vi "GET CUSTOM ITEM.vi"(11 "REFERENCES":T1) -> ()   [LabVIEW 2019]
uses:
  Controls/References Cluster.ctl
  <vilib>/userDefined/High Color/IMAQdx.ctl
  Controls/Custom Calendar/Custom Calendar.xctl
types:
  T1 = typedef "References Cluster.ctl" = cluster{"MAIN PAGES":refnum<vi>, "ADD/EDIT ITEM REFERENCES":cluster{"Identifier":refnum<vi>, "BYU ICN #":refnum<vi>, "Item Description":refnum<vi>, "Comments":refnum<vi>, "Checked Out Date":refnum<vi>, "Due Date":refnum<vi>, "Check Out Location":refnum<vi>, "Reminder Count":refnum<vi>, "Most Recent Reminder Date":refnum<vi>, "BYU ID #":refnum<vi>, "Building/Room":refnum<vi>, "Location in Room":refnum<vi>, "Manual":refnum<vi>, "Manufacturer":refnum<vi>, "Model #":refnum<vi>, "Serial #":refnum<vi>, "Date Acquired":refnum<vi>, "ADD/EDIT ITEM LABEL":refnum<vi>, "ARCHIVE ITEM":refnum<vi>, "Archive Item Inputs":refnum<vi>, "Reminder Notes":refnum<vi>}, "ADD/EDIT USER REFERENCES":cluster{"BYU ID # (##-###-####)":refnum<vi>, "First Name":refnum<vi>, "Last Name":refnum<vi>, "Phone Number (###-###-####)":refnum<vi>, "Email":refnum<vi>, "Department":refnum<vi>, "Graduation Status":refnum<vi>, "Anticipated Graduation Year":refnum<vi>, "Credit Score":refnum<vi>, "Date Added":refnum<vi>, "Graduation Clearance Date":refnum<vi>, "Picture File Name":refnum<vi>, "ADD/EDIT USER LABEL":refnum<vi>, "Department Map":refnum<vi>, "Status Map":refnum<vi>, "Anticipated Graduation Year Map":refnum<vi>, "User Agreement":refnum<vi>, "User Comments":refnum<vi>, "Camera":refnum<vi>}, "RETURN ITEM REFERENCES":cluster{"Item or Person:":refnum<vi>, "Search Return Results":refnum<vi>, "What are you searching for?":refnum<vi>}, "SEARCH DATABASE REFERENCES":cluster{"What to Search For:":refnum<vi>, "Where to Search":refnum<vi>, "Column to Search In":refnum<vi>, "Column to Sort By":refnum<vi>, "Search Database Results":refnum<vi>, "Inventory Column Selector":refnum<vi>, "User Column Selector":refnum<vi>, "Inventory Archive Column Selector":refnum<vi>, "User Archive Column Selector":refnum<vi>, "Sales Tracking Column Selector":refnum<vi>, "Checked In Archive Column Selector":refnum<vi>, "Restore User":refnum<vi>, "Date Range":refnum<vi>, "Dates Less Than":refnum<vi>, "Dates Greater Than":refnum<vi>, "Search Print Receipt":refnum<vi>, "Edit Sale Description":refnum<vi>}, "USER ITEMS REFERENCES":cluster{"USER'S INFORMATION":refnum<vi>, "User's Checked Out Items":refnum<vi>, "User Info Comments":refnum<vi>, "SEE USER INFO COMMENTS":refnum<vi>}, "EDIT ITEMS REFERENCES":cluster{"New Check Out Location":refnum<vi>, "Items to Edit":refnum<vi>, "Edit Items Due Date":refnum<vi>, "New Reminder Notes":refnum<vi>, "New Item Description":refnum<vi>}, "CHECK OUT ITEMS REFERENCES":cluster{"Enter Item:":refnum<vi>, "Check Out Items Due Date":refnum<vi>, "Check Out Location":refnum<vi>, "Items to be Checked Out":refnum<vi>, "Possible Items":refnum<vi>}, "TRANSFER ITEMS REFERENCES":cluster{"Search Parameter":refnum<vi>, "What to Match":refnum<vi>, "Matching Individuals":refnum<vi>, "Items to be Transferred":refnum<vi>}, "SETTINGS REFERENCES":cluster{"PSC Database Settings":refnum<vi>, "PSC Sales Item Spreadsheet":refnum<vi>}, "PSC SALES REFERENCES":cluster{"BYU ID CARD #":refnum<vi>, "Sale Description":refnum<vi>, "Scan or Enter Item Name":refnum<vi>, "Items to be Sold":refnum<vi>, "Grand Total":refnum<vi>, "Item List":refnum<vi>}}
  T2 = cluster{"BYU ID CARD #":refnum<vi>, "Sale Description":refnum<vi>, "Scan or Enter Item Name":refnum<vi>, "Items to be Sold":refnum<vi>, "Grand Total":refnum<vi>, "Item List":refnum<vi>}
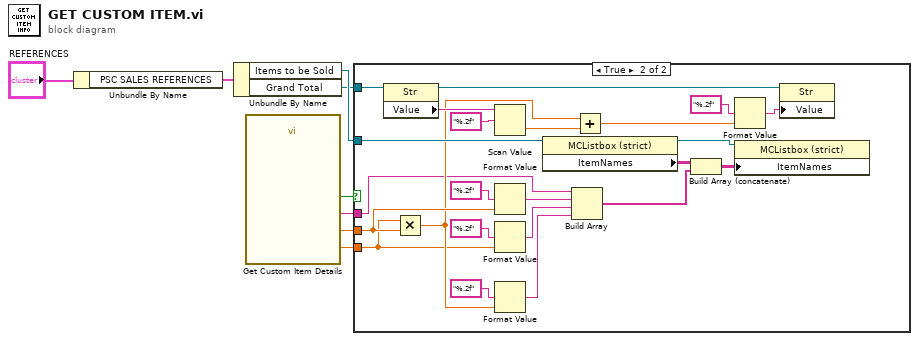
[diagram p0: block diagram]
diagram:
  n1 = Unbundle By Name("REFERENCES") -> ("PSC SALES REFERENCES"=w7:T2)
  n2 = Unbundle By Name(w7) -> ("Items to be Sold"=w5:refnum<vi>, "Grand Total"=w4:refnum<vi>)
  n3 = call "Get Custom Item Details"() -> ("Price"=w1:dbl, "Quantity"=w3:dbl, "Name"=w2:string, "OK"=w6:bool)  [unwired: 15 in, 1 out]
  n4 = case shown="True" w6 {
    tunnel: w3 -> [_ w26]
    tunnel: w5 -> [_ w31]
    tunnel: w4 -> [_ w30]
    tunnel: w2 -> [_ w12]
    tunnel: w1 -> [_ w11]
    frame False {
    }
    frame True {
      n5 = property class="Str"(reference=w30) -> (reference out=w20:refnum<vi>, "Value"=w24:string)  [unwired: 1 in, 1 out]
      n6 = Multiply(x=w11, y=w26) -> (x*y=w13:dbl)
      n7 = Scan Value(string=w24, format string="%.2f") -> (value=w23:dbl)  [unwired: 1 in, 1 out]
      n8 = Format Value(format string="%.2f", value (0)=w26) -> (output string=w27:string)  [unwired: 1 in]
      n9 = Format Value(format string="%.2f", value (0)=w11) -> (output string=w9:string)  [unwired: 1 in]
      n10 = Format Value(format string="%.2f", value (0)=w13) -> (output string=w17:string)  [unwired: 1 in]
      n11 = property class="MCListbox (strict)"(reference=w31) -> (reference out=w15:refnum<vi>, "ItemNames"=w29:string[][])  [unwired: 1 in, 1 out]
      n12 = Build Array(w12, w27, w9, w17) -> (w16:string[])
      n13 = Add(x=w13, y=w23) -> (x+y=w21:dbl)
      n14 = Build Array (concatenate)(w29, w16) -> (w14:string[][])
      n15 = Format Value(format string="%.2f", value (0)=w21) -> (output string=w19:string)  [unwired: 1 in]
      n16 = property class="MCListbox (strict)"(reference=w15, "ItemNames"=w14) -> ()  [unwired: 1 in, 2 out]
      n17 = property class="Str"(reference=w20, "Value"=w19) -> ()  [unwired: 1 in, 2 out]
    }
  }
